vi "Installer Set Product Version__icon_lib_labview_project_api.vi"(8 "error in (no error)":errorcluster, 10 "Installer Version":string, 11 "Build Spec Reference":refnum<vi>) -> (0 "error out":errorcluster, 3 "Build Spec Reference Dup":refnum<vi>)   [LabVIEW 2013, in "LabVIEW Project API__icon_lib_labview_project_api.lvlib"]
doc: "Sets the Product Version for an Installer Build Specification.\n\nE.g. \"1.0.0\"\n\n<b>Author:</b> JG\n\n<b>ICON Technologies Pty Ltd</b>\nCopyright (C) 1990-2009\nAll Rights Reserved"
uses:
  LabVIEW Project API__icon_lib_labview_project_api.lvlib
panel:
  # "Output"
  # "Input"
  # "ICON Technologies Pty Ltd\nCopyright (C) 1990-2009\nAll Rights Reserved"
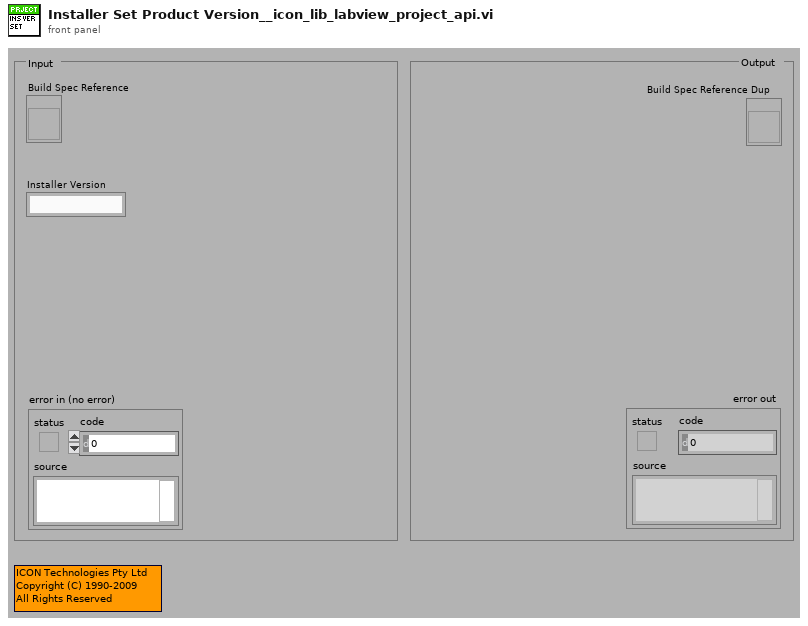
[diagram p1: front panel]
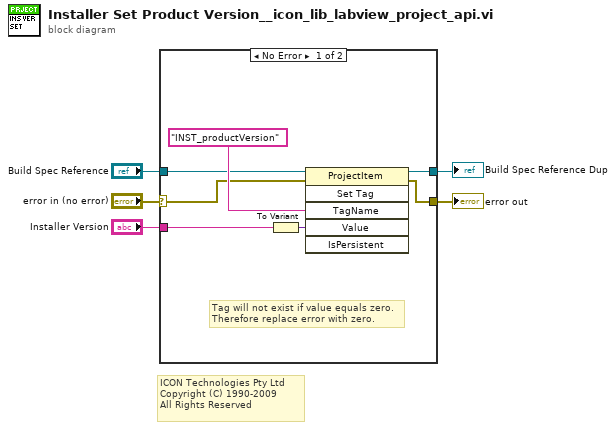
[diagram p0: block diagram]
diagram:
  # "ICON Technologies Pty Ltd\nCopyright (C) 1990-2009\nAll Rights Reserved"
  n1 = case shown="No Error" "error in (no error)" {
    selector: "error in (no error)" -> [w7 w14]
    tunnel: [w9 w14] -> w4
    tunnel: "Build Spec Reference" -> [w8 w13]
    tunnel: [w10 w13] -> w2
    tunnel: "Installer Version" -> [w6 _]
    frame No Error {
      # "Tag will not exist if value equals zero.\nTherefore replace error with zero."
      n2 = To Variant(anything=w6) -> (Variant=w11:variant)
      n3 = invoke class="ProjectItem" method="Set Tag"(reference=w8, error in=w7, "TagName"="INST_productVersion" ("Tag Name"), "Value"=w11) -> (reference out=w10:refnum<vi>, error out=w9:errorcluster)  [unwired: 2 in, 4 out]
    }
    frame Error {
    }
  }
  "error out" <- w4
  "Build Spec Reference Dup" <- w2
